vi "Generate Pitch Waveform.vi"() -> (0 "Error Out":errorcluster, 3 "Y":dbl[](array[numeric]))   [LabVIEW 2014]
uses:
  <vilib>/measure/NI_MABase.lvlib
panel:
  in  "sampling info":cluster{"Fs":dbl, "#s":dbl}={"Fs"=1000.0, "#s"=1000.0} {"Fs" format="%.2p"}
  in  "frequency":dbl=10.0 format="%0.2p"
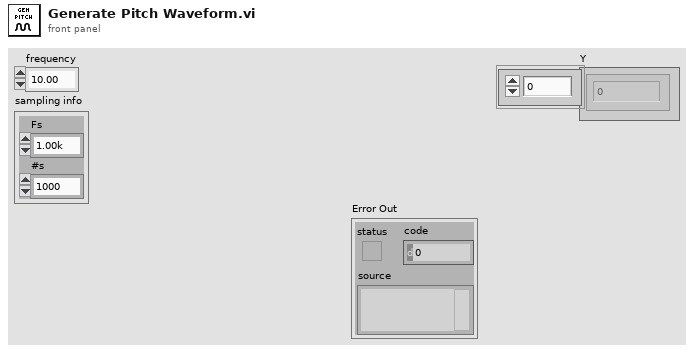
[diagram p1: front panel]
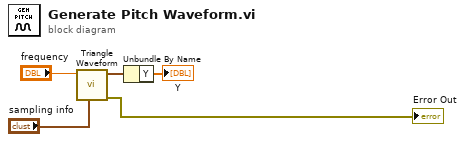
[diagram p0: block diagram]
diagram:
  n1 = call <vilib>:"Triangle Waveform.vi"("sampling info"="sampling info", "frequency"="frequency") -> ("error out"=→"Error Out":errorcluster, "signal out"=w4:waveform(dbl))  [unwired: 8 in]
  n2 = Unbundle By Name(w4) -> ("Y"=→"Y":dbl[])
